vi "Initialize.vi"(8 "error in (no error)":errorcluster, 11 "UI in":refnum<class "UI.lvclass">) -> (0 "error out":errorcluster, 3 "UI out":refnum<class "UI.lvclass">, 4 "UI Event Registrations":T1)   [LabVIEW 2020, in "AR Example.lvlib" / "UI.lvclass"]
uses:
  UI.lvclass
  Stop Event.ctl
  Events.ctl
  Update Preview Event.ctl
  g_ar_toolkit.image/Image Draw Offset.ctl
  Popup Image Window.vi
  Popup Image Window Action.ctl
  Popup Image Window Events.ctl
  UI Event Registrations.ctl
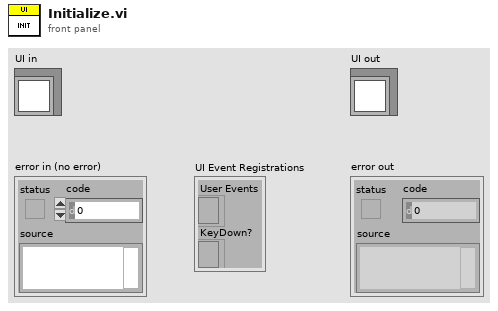
[diagram p1: front panel]
types:
  T1 = typedef "AR Example.lvlib/UI.lvclass/UI Event Registrations.ctl" = cluster{"User Events":refnum<event-registration>, "KeyDown?":refnum<event-registration>}
  T2 = typedef "AR Example.lvlib/UI.lvclass/Update Preview Event.ctl" = cluster{"Image":refnum<data-value>, "Draw Offset":T3}
  T3 = typedef "g_ar_toolkit.image.lvlib/Image Draw Offset.ctl" = cluster{"Left":i16, "Top":i16}
  T4 = typedef "AR Example.lvlib/UI.lvclass/Popup Image Window Events.ctl" = cluster{"Update Image":refnum<user-event>, "Action":refnum<user-event>, "Update Window Name":refnum<user-event>}
  T5 = typedef "AR Example.lvlib/UI.lvclass/Events.ctl" = cluster{"Stop":refnum<user-event>, "Camera Setup Display":refnum<user-event>, "Camera Cal Display":refnum<user-event>, "Enable Disable Key Events":refnum<user-event>}
  T6 = typedef "AR Example.lvlib/UI.lvclass/Stop Event.ctl" = cluster{"Data":bool}
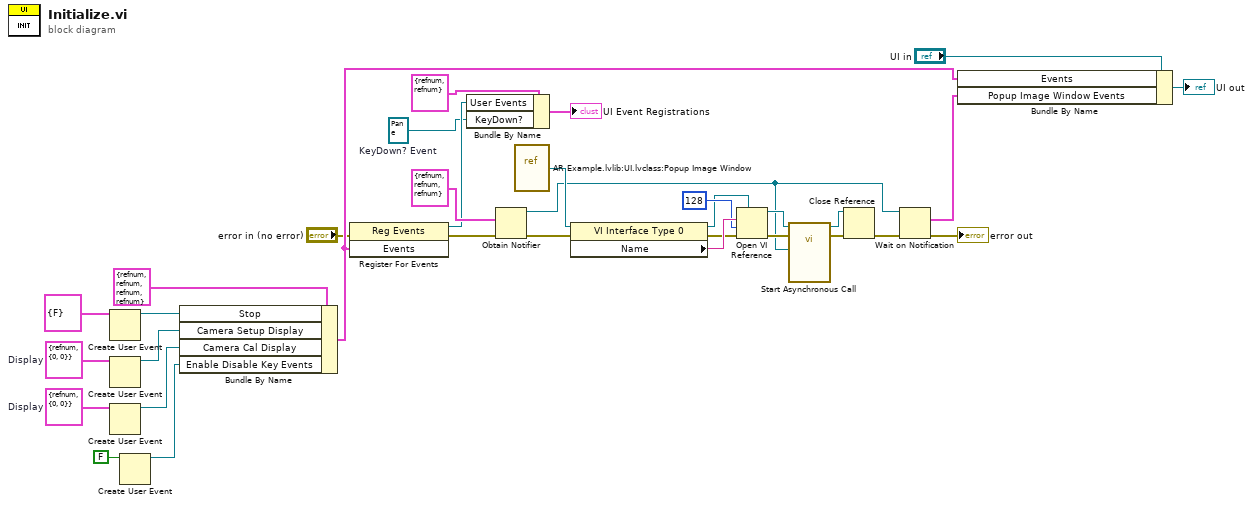
[diagram p0: block diagram]
diagram:
  w3 = refnum<event-registration> refnum  # KeyDown? Event
  w8 = T2 {"Image"=refnum, "Draw Offset"={"Left"=0, "Top"=0}}  # Display
  w28 = T2 {"Image"=refnum, "Draw Offset"={"Left"=0, "Top"=0}}  # Display
  n1 = Create User Event(user event datatype=T6 {"Data"=FALSE} ("Stop")) -> (user event=w31:refnum<user-event>)  [unwired: 1 in, 1 out]
  n2 = Create User Event(user event datatype=w28) -> (user event=w26:refnum<user-event>)  [unwired: 1 in, 1 out]
  n3 = Create User Event(user event datatype=w8) -> (user event=w9:refnum<user-event>)  [unwired: 1 in, 1 out]
  n4 = Create User Event(user event datatype=FALSE ("Enable/Disable")) -> (user event=w5:refnum<user-event>)  [unwired: 1 in, 1 out]
  n5 = Bundle By Name(cluster=T5 {"Stop"=refnum, "Camera Setup Display"=refnum, "Camera Cal Display"=refnum, "Enable Disable Key Events"=refnum} ("Events"), "Stop"=w31, "Camera Setup Display"=w26, "Camera Cal Display"=w9, "Enable Disable Key Events"=w5) -> (w29:T5)
  n6 = register-events(error in="error in (no error)", w29) -> (reference out=w4:refnum<event-registration>, error out=w13:errorcluster)  [unwired: 1 in]
  n7 = Bundle By Name(cluster=T1 {"User Events"=refnum, "KeyDown?"=refnum} ("UI Event Registrations"), "User Events"=w4, "KeyDown?"=w3) -> (→"UI Event Registrations":T1)
  n8 = Obtain Notifier(notification data type=T4 {"Update Image"=refnum, "Action"=refnum, "Update Window Name"=refnum} ("Popup Image Window Events"), error in (no error)=w13) -> (notifier out=w11:refnum<notifier>, error out=w14:errorcluster)  [unwired: 2 in, 1 out]
  n9 = vi-ref "AR Example.lvlib:UI.lvclass:Popup Image Window.vi"() -> (w25:refnum<vi>)
  n10 = property class="VI Interface Type 0"(reference=w25, error in=w14) -> (reference out=w21:refnum<vi>, error out=w23:errorcluster, "Name"=w24:string)
  n11 = Open VI Reference(type specifier VI Refnum (for type only)=w21, vi path=w24, options=128, error in (no error)=w23) -> (vi reference=w20:refnum<vi>, error out=w19:errorcluster)  [unwired: 2 in]
  n12 = call-by-ref "Start Asynchronous Call"(reference=w20, error in=w19, "Event Passback"=w11) -> (reference out=w17:refnum<vi>, error out=w16:errorcluster)  [unwired: 11 in]
  n13 = Close Reference(reference=w17, error in (no error)=w16) -> (error out=w12:errorcluster)
  n14 = Wait on Notification(notifier=w11, error in (no error)=w12) -> (notification=w7:T4, error out=→"error out":errorcluster)  [unwired: 2 in, 2 out]
  n15 = Bundle By Name(cluster="UI in", "Events"=w29, "Popup Image Window Events"=w7) -> (→"UI out":refnum<class "UI.lvclass">)
